vi "Create_Default_Destinations.vi"(8 "error in (no error)":errorcluster, 9 "Destination Name":string, 10 "Destination Path":path, 11 "AB_PackedLibrary in":refnum<class "AB_PackedLibrary.lvclass">) -> (0 "error out":errorcluster, 2 "default dests":refnum<class "AB_Destination.lvclass">[](array[class]), 3 "AB_PackedLibrary out":refnum<class "AB_PackedLibrary.lvclass">)   [LabVIEW 2020, in "AB_PackedLibrary.lvclass"]
uses:
  <vilib>/AppBuilder/AB_Classes/PackedLib/AB_PackedLibrary.lvclass
  <vilib>/AppBuilder/AB_Classes/Destination/AB_Destination.lvclass
  <vilib>/AppBuilder/AB_Classes/Destination/Dest_Application/AB_Dest_App.lvclass
  e:/builds/penguin/labview/branches/2020/dev/dist/vi.lib/AppBuilder/AB_Classes/Destination/AB_Destination.lvclass
  <vilib>/AppBuilder/AB_Classes/Destination/AB_Destination.ctl
  <resource>/Framework/Providers/Common/provcom_StringGlobals.vi
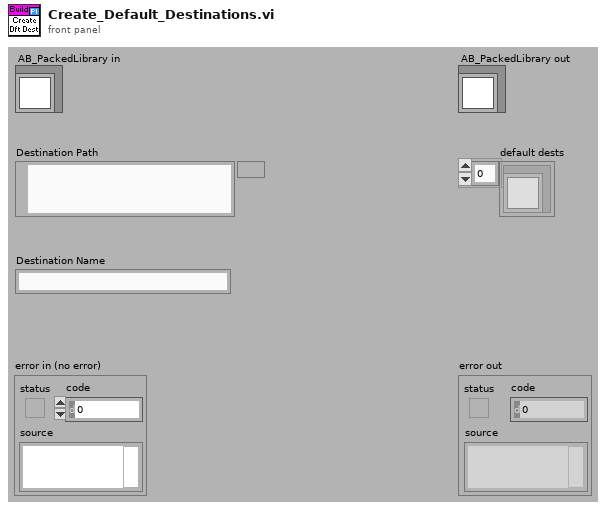
[diagram p1: front panel]
types:
  T1 = typedef "AB_Destination.ctl" = cluster{"destName":string, "path":path, "libraryName":string, "preserveHierarchy":bool, "eng_inBuild":bool, "eng_libraryReference":refnum<vi>, "eng_restictAddToNewLibrary":bool}
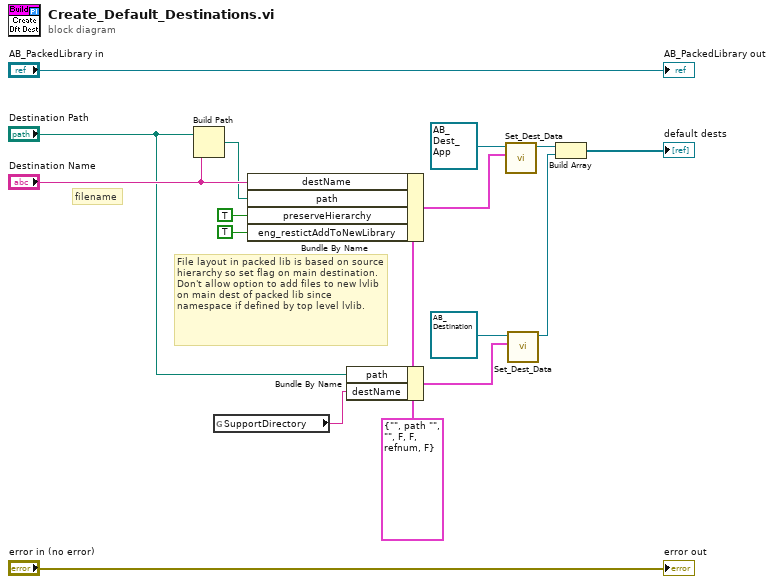
[diagram p0: block diagram]
diagram:
  w10 = T1 {"destName"="", "path"=path "", "libraryName"="", "preserveHierarchy"=FALSE, "eng_inBuild"=FALSE, "eng_libraryReference"=refnum, "eng_restictAddToNewLibrary"=FALSE} ("destName")
  # "filename"
  # "File layout in packed lib is based on source hierarchy so set flag on main destination.\nDon't allow option to add files to new lvlib on main dest of packed lib since namespace if defined by top level lvlib."
  n1 = Build Path(base path="Destination Path", name or relative path="Destination Name") -> (appended path=w4:path)
  n2 = global read "provcom_StringGlobals.vi" "SupportDirectory"() -> (w12:string)
  n3 = Bundle By Name(cluster=w10, "destName"="Destination Name", "path"=w4, "preserveHierarchy"=TRUE, "eng_restictAddToNewLibrary"=TRUE ("eng_restictAddToLibrary")) -> (w15:T1)
  n4 = Bundle By Name(cluster=w10, "path"="Destination Path", "destName"=w12) -> (w13:T1)
  n5 = call <vilib>:"Set_Dest_Data.vi"("destName"=w15, "Class in"=refnum<class "AB_Dest_App.lvclass"> refnum ("AB_Dest_App.lvclass")) -> ("Class out"=w16:refnum<class "AB_Dest_App.lvclass">)  [unwired: 1 in, 8 out]
  n6 = call <vilib>:"Set_Dest_Data.vi"("destName"=w13, "Class in"=refnum<class "AB_Destination.lvclass"> refnum ("AB_Destination.lvclass")) -> ("Class out"=w14:refnum<class "AB_Destination.lvclass">)  [unwired: 1 in, 8 out]
  n7 = Build Array(w16, w14) -> (→"default dests":refnum<class "AB_Destination.lvclass">[])
  "error out" <- "error in (no error)"
  "AB_PackedLibrary out" <- "AB_PackedLibrary in"
